vi "Python_Logic2_Automation.vi"() -> ()   [LabVIEW 2023]
doc: "This example demonstrates how to use Python to control the Ssaleae Logic2 software supporting the Logic 8, Logic Pro 8 and Logic Pro 16 logic annalyzers."
uses:
  <vilib>/Utility/sysdir.llb/System Directory Type.ctl
  <vilib>/Python/Open Anaconda Python Session.vi
panel:
  in  "Save Data?":bool
  out "Saleae Capture":string
  out "Raw Digital":string
  out "SPI Analyzer":string
  in  "Analyzer Settings":T1={"MOSI Channel"=0, "MISO Channel"=1, "CLOCK Channel"=2, "ENABLE Channel"=3, "Bits per Transfer"="8 Bits per Transfer (Standard)"}
  in  "Analyzer Label":string="Test Analyzer"
  in  "Digital Config":T2={"Enabled Digital Channels"=[0, 1, 2, 3], "Digital Sample Rate (Samp/Sec)"=10000000, "Digital Threshold(V)"=3.3000000000000007} {"Digital Threshold(V)" format="%#_13g"; "Digital Sample Rate (Samp/Sec)" format="%.0p"}
  in  "Device ID":string="F4241"
  in  "Capture Duration (s)":dbl=5.0 format="%#_13g"
  in  "Port [10430]":i32=10430
  in  "IP Address [127.0.0.1]":string="127.0.0.1"
  out "Anaconda3 Path":path
  in  "Python version":string="3.8"
  in  "Anaconda Environment":string="Python38"
  out "error out":errorcluster
  in  "error in (no error)":errorcluster
  # "1. Python Settings"
  # "2. Logic2 Automation Server"
  # "3. Configure Device"
  # "4. Configure Capture"
  # "5. Start Capture"
  # "6. Add SPI Analyzer"
  # "7. Saved Files"
  # "Overview: Demonstrates how to use Python to automate the Saleae Logic2 software.\nRequirements: Python 3.8, 3.9 or 3.10 with the same bitness as LabVIEW.\nInstructions:\n1. Install LabVIEW, and setup an Anaconda 3 instance using Python 3.8\n  https://knowledge.ni.com/KnowledgeArticleDetails?id=kA00Z0000015C6tSAE&l=en-US \n2. Install the Saleae Python library using the instructions found here:\n  https://saleae.github.io/logic2-automation/getting_started.html#installing-the-python-automation-api-package\n# 3. Be sure Automation is enabled in the Logic2 Software (Saleae link above)\n# 4. The key parameters in this VI are the Anaconda setup and the Saleae 'Device ID' (F4241 is the default simulated Logic Pro 16)"
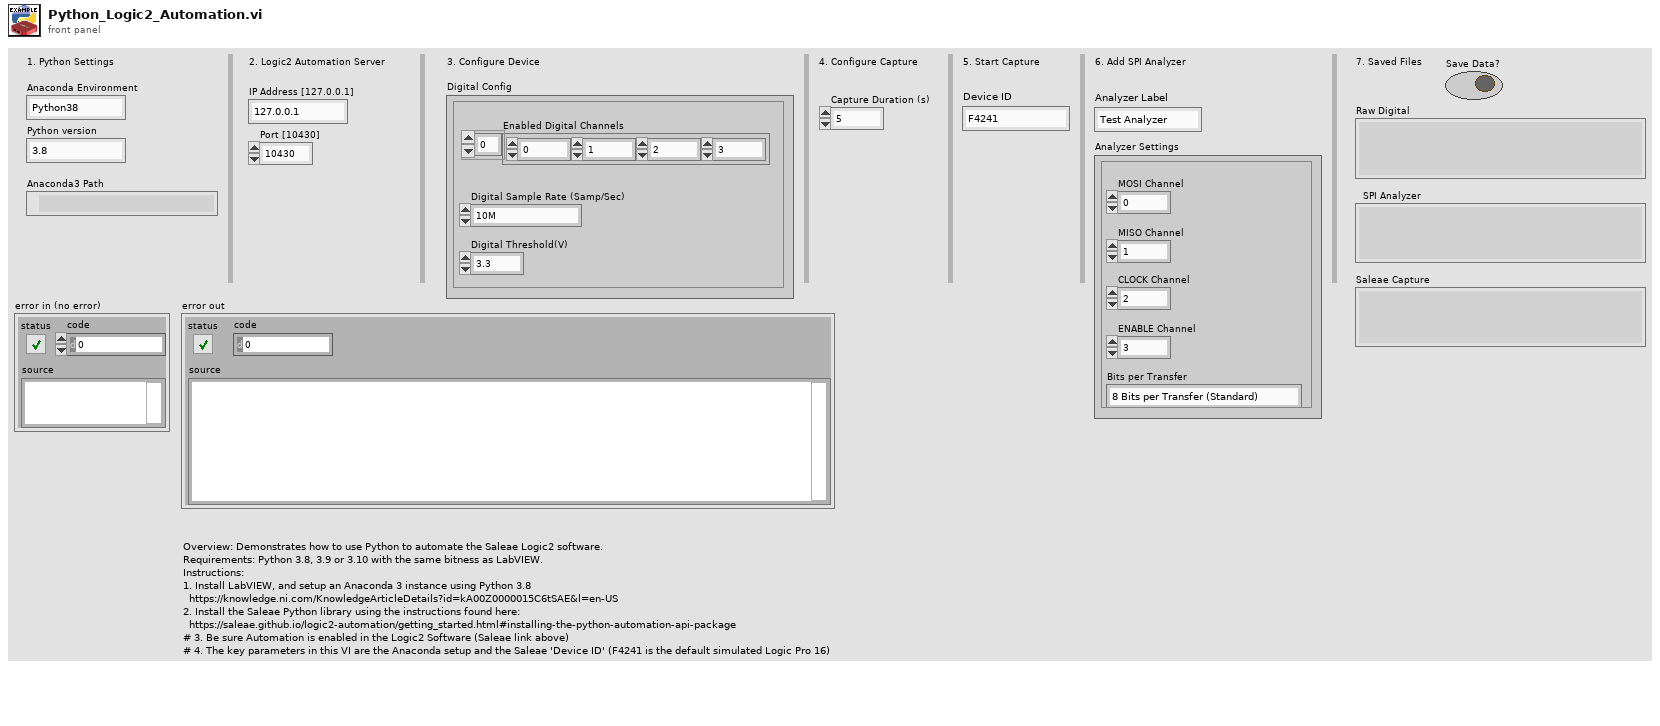
[diagram p1: front panel]
types:
  T1 = cluster{"MOSI Channel":i32, "MISO Channel":i32, "CLOCK Channel":i32, "ENABLE Channel":i32, "Bits per Transfer":string}
  T2 = cluster{"Enabled Digital Channels":i32[], "Digital Sample Rate (Samp/Sec)":i32, "Digital Threshold(V)":dbl}
  T3 = typedef "System Directory Type.ctl" = i32
  T4 = cluster{"Refnum in":refnum<k35>, "Python Module Name":path}
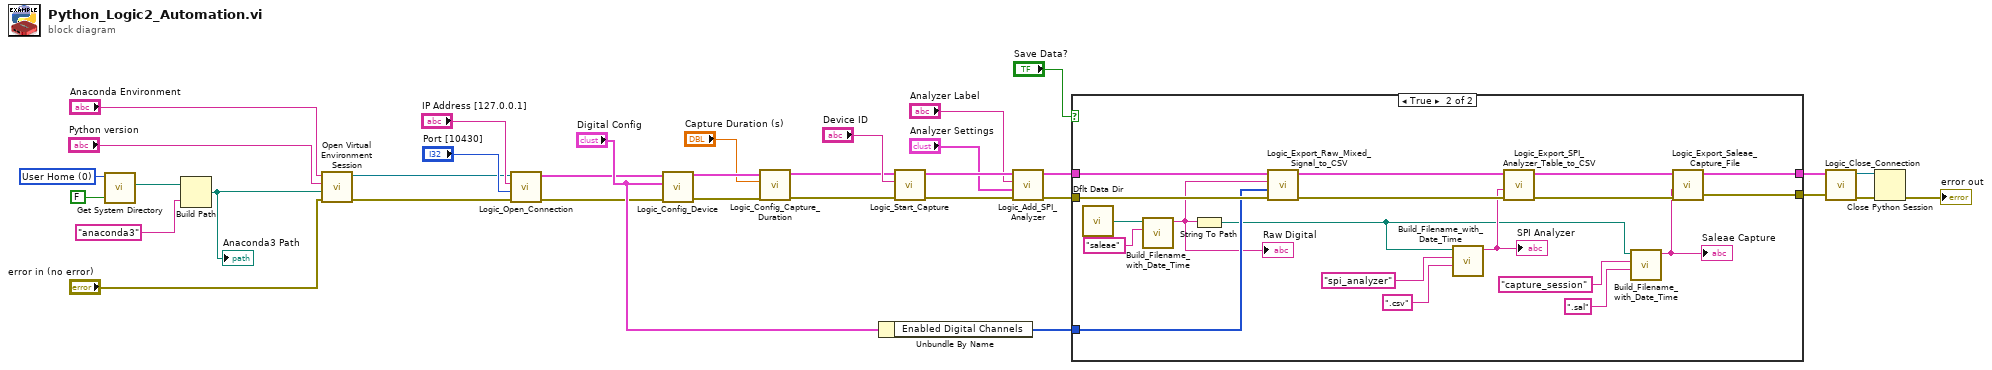
[diagram p0: block diagram]
diagram:
  w28 = T3 0 items=["User Home"=0, "User Desktop"=1, "User Documents"=2, "User Application Data"=3, "User Preferences"=4, "User Temporary"=5, "Public Documents"=6, "Public Application Data"=7, "Public Preferences"=8, "Public Cache"=13, "System Core Libraries"=9, "System Installed Libraries"=10, "Application Files"=11, "Boot Volume Root"=12] ("system directory type")
  n1 = call <vilib>:"Get System Directory.vi"("create directory if not found? (F)"=FALSE, "system directory type"=w28) -> ("system directory"=w26:path)  [unwired: 9 in]
  n2 = Build Path(base path=w26, name or relative path="anaconda3") -> (appended path=w29:path)
  "Anaconda3 Path" <- w29
  n3 = call-poly <vilib>:"Open Virtual Environment Session.vi"("error in (no error)"="error in (no error)", "Anaconda path"=w29, "Python version"="Python version", "Env name"="Anaconda Environment") -> ("error out"=w13:errorcluster, "session out"=w14:refnum<k35>)  [unwired: 6 in]
  n4 = call "Logic_Open_Connection.vi"("error in (no error)"=w13, "Port [10430]"="Port [10430]", "IP Address [127.0.0.1]"="IP Address [127.0.0.1]", "Python Session In"=w14) -> ("error out"=w9:errorcluster, "Session Ref Out"=w17:T4)  [unwired: 1 in, 1 out]
  n5 = call "Logic_Config_Device.vi"("error in (no error)"=w9, "Digital Config"="Digital Config", "Session Ref In"=w17) -> ("error out"=w18:errorcluster, "Session Ref Out"=w21:T4)  [unwired: 2 in, 1 out]
  n6 = call "Logic_Config_Capture_Duration.vi"("error in (no error)"=w18, "Capture Duration (s)"="Capture Duration (s)", "Session Ref In"=w21) -> ("error out"=w19:errorcluster, "Session Ref Out"=w22:T4)  [unwired: 2 in, 1 out]
  n7 = Unbundle By Name("Digital Config") -> ("Enabled Digital Channels"=w4:i32[])
  n8 = call "Logic_Start_Capture.vi"("error in (no error)"=w19, "Device ID"="Device ID", "Session Ref In"=w22) -> ("error out"=w23:errorcluster, "Session Ref Out"=w24:T4)  [unwired: 2 in, 1 out]
  n9 = call "Logic_Add_SPI_Analyzer.vi"("error in (no error)"=w23, "Analyzer Settings"="Analyzer Settings", "Analyzer Label"="Analyzer Label", "Session Ref In"=w24) -> ("error out"=w6:errorcluster, "Session Ref Out"=w5:T4)  [unwired: 1 in, 1 out]
  n10 = case shown="True" "Save Data?" {
    tunnel: w6 -> [w35 w55]
    tunnel: w5 -> [w36 w54]
    tunnel: w4 -> [_ w53]
    tunnel: [w36 w43] -> w3
    tunnel: [w35 w42] -> w2
    frame False {
    }
    frame True {
      n11 = call <vilib>:"Dflt Data Dir.vi"() -> ("App:Default Data Directory"=w40:path)
      n12 = call "Build_Filename_with_Date_Time.vi"("Item Prefix"="saleae" ("Filename Prefx"), "Folder for Data Captures"=w40) -> ("File Path Output"=w37:string)  [unwired: 9 in]
      "Raw Digital" <- w37
      n13 = String To Path(string=w37) -> (path=w38:path)
      n14 = call "Logic_Export_Raw_Mixed_Signal_to_CSV.vi"("error in (no error)"=w55, "Enabled Digital Channels"=w53, "Filepath Input"=w37, "Session Ref In"=w54) -> ("error out"=w51:errorcluster, "Session Ref Out"=w52:T4)  [unwired: 5 in, 1 out]
      n15 = call "Build_Filename_with_Date_Time.vi"("File Extension (.csv)"=".csv", "Item Prefix"="spi_analyzer" ("Filename Prefx"), "Folder for Data Captures"=w38) -> ("File Path Output"=w46:string)  [unwired: 8 in]
      "SPI Analyzer" <- w46
      n16 = call "Logic_Export_SPI_Analyzer_Table_to_CSV.vi"("error in (no error)"=w51, "Filepath Input"=w46, "Session Ref In"=w52) -> ("error out"=w47:errorcluster, "Session Ref Out"=w48:T4)  [unwired: 2 in, 1 out]
      n17 = call "Build_Filename_with_Date_Time.vi"("File Extension (.csv)"=".sal", "Item Prefix"="capture_session" ("Filename Prefx"), "Folder for Data Captures"=w38) -> ("File Path Output"=w41:string)  [unwired: 8 in]
      "Saleae Capture" <- w41
      n18 = call "Logic_Export_Saleae_Capture_File.vi"("error in (no error)"=w47, "Filepath Input"=w41, "Session Ref In"=w48) -> ("error out"=w42:errorcluster, "Session Ref Out"=w43:T4)  [unwired: 2 in, 1 out]
    }
  }
  n19 = call "Logic_Close_Connection.vi"("error in (no error)"=w2, "Session Ref In"=w3) -> ("error out"=w7:errorcluster, "Python Session Out"=w8:refnum<k35>)  [unwired: 3 in, 1 out]
  n20 = Close Python Session(session in=w8, error in=w7) -> (11:→"error out":errorcluster)
